vi "FTW-JSON-Core-ElementType.vi"(1 "Core Type":T2=enum."undefined") -> (0 "JSON Element Type":T1)   [LabVIEW 2014]
uses:
  FTW-JSON-Core-Type.ctl
  FTW-JSON-Type.ctl
panel:
  # "Inputs"
  # "Outputs"
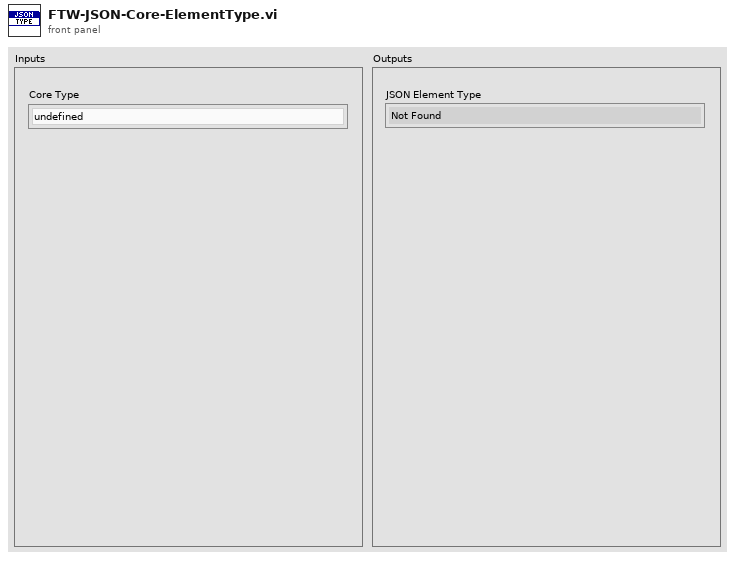
[diagram p1: front panel]
types:
  T1 = typedef "FTW-JSON-Type.ctl" = enum8{"Not Found", "Object", "Array", "String", "Number", "Boolean", "null"}
  T2 = typedef "FTW-JSON-Core-Type.ctl" = enum8{"Object", "Array", "String", "Integer", "Floating Point", "true", "false", "null", "undefined"}
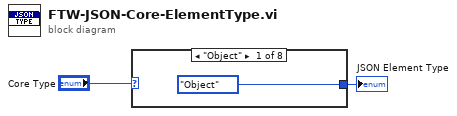
[diagram p0: block diagram]
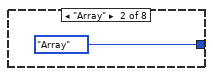
[diagram p2: hidden frame]
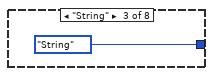
[diagram p3: hidden frame]
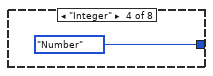
[diagram p4: hidden frame]
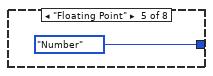
[diagram p5: hidden frame]
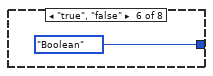
[diagram p6: hidden frame]
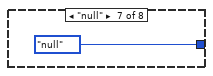
[diagram p7: hidden frame]
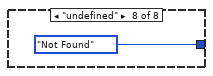
[diagram p8: hidden frame]
diagram:
  n1 = case shown="\"Object\"" "Core Type" {
    tunnel: [FTW-JSON-Type."Object" FTW-JSON-Type."Array" FTW-JSON-Type."String" FTW-JSON-Type."Number" FTW-JSON-Type."Number" FTW-JSON-Type."Boolean" FTW-JSON-Type."null" FTW-JSON-Type."Not Found"] -> w1
    frame "Object" {
    }
    frame "Array" {
    }
    frame "String" {
    }
    frame "Integer" {
    }
    frame "Floating Point" {
    }
    frame "true", "false" {
    }
    frame "null" {
    }
    frame "undefined" {
    }
  }
  "JSON Element Type" <- w1
